vi "setUp.vi"(8 "error in (no error)":errorcluster, 11 "reference in":refnum<class "testcase-CSMNonCSMCallerSupportAPI.lvclass">) -> (0 "error out":errorcluster, 3 "reference out":refnum<class "testcase-CSMNonCSMCallerSupportAPI.lvclass">)   [LabVIEW 2017, in "testcase-CSMNonCSMCallerSupportAPI.lvclass"]
doc: "setUp runs prior to the test method during test execution. Use this method to initialize any object data required by your tests."
uses:
  testcase-CSMNonCSMCallerSupportAPI.lvclass
  C:/Program Files (x86)/National Instruments/LabVIEW 2017/vi.lib/addons/_JKI Toolkits/VI Tester/TestCase.llb/TestCase.lvclass
  testcase-CSMNonCSMCallerSupportAPI.lvclass/testcase-CSMNonCSMCallerSupportAPI.ctl
  <vilib>/addons/_JKI Toolkits/VI Tester/TestCase.llb/TestCase.lvclass
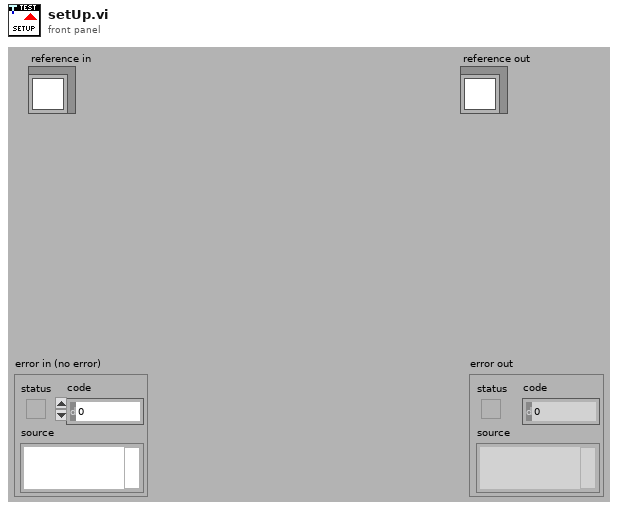
[diagram p1: front panel]
types:
  T1 = cluster{"name":string, "num":i32, "prototype":string[]}[]
  T2 = cluster{"prototype":string, "name":string, "num":i32, "index":i32}[]
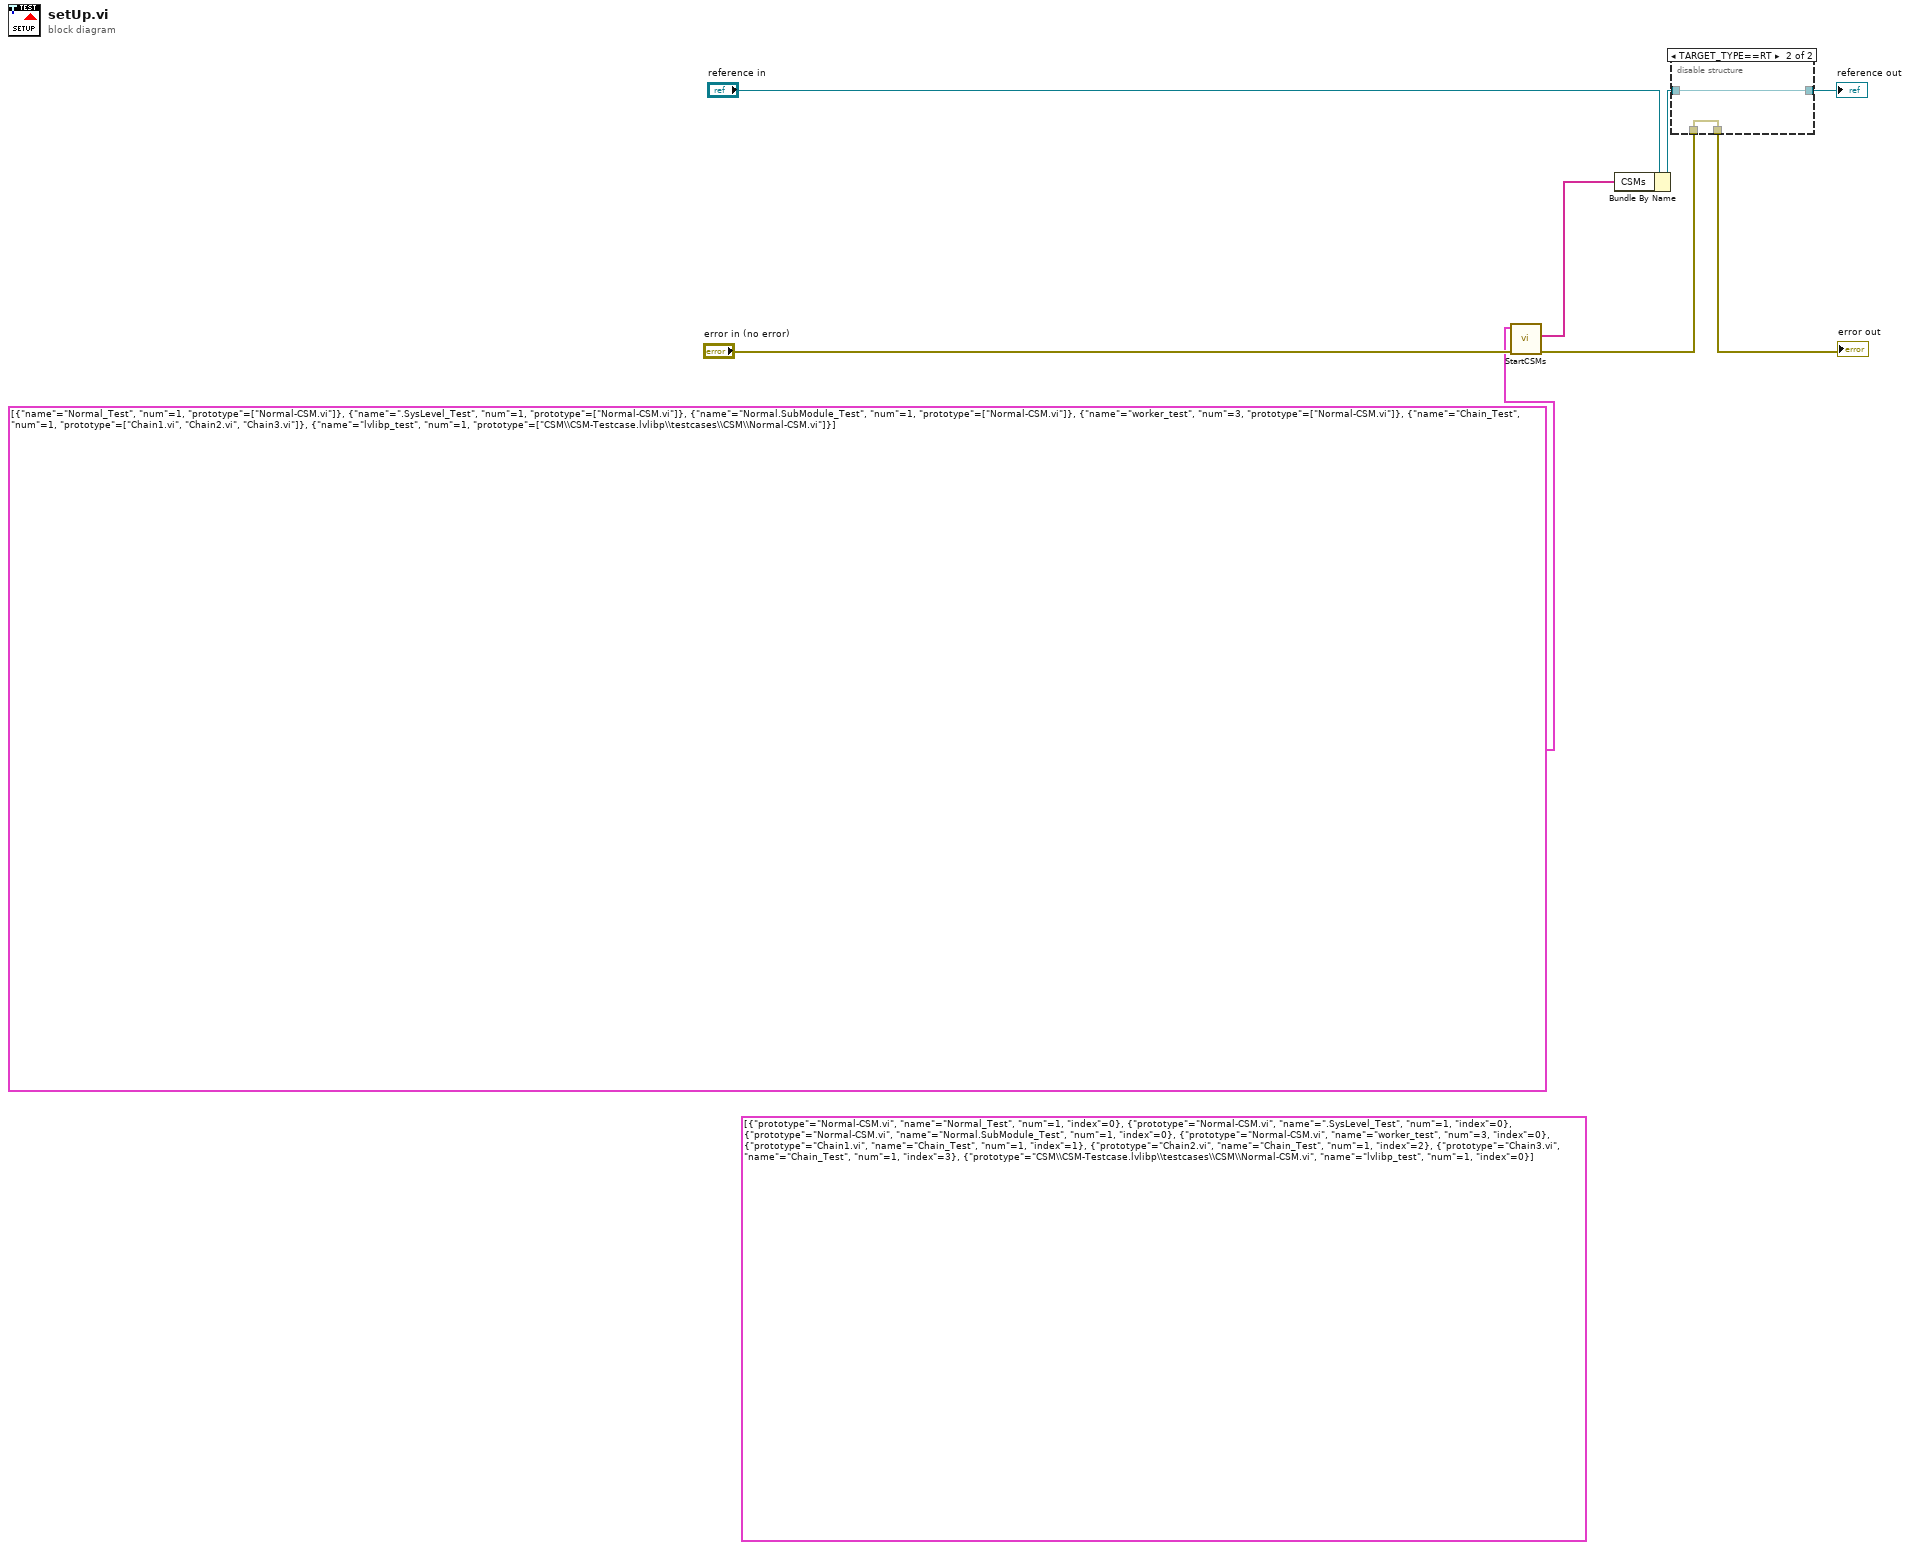
[diagram p0: block diagram]
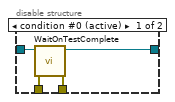
[diagram p2: hidden frame]
diagram:
  (unwired) T2 [{"prototype"="Normal-CSM.vi", "name"="Normal_Test", "num"=1, "index"=0}, {"prototype"="Normal-CSM.vi", "name"=".SysLevel_Test", "num"=1, "index"=0}, {"prototype"="Normal-CSM.vi", "name"="Normal.SubModule_Test", "num"=1, "index"=0}, {"prototype"="Normal-CSM.vi", "name"="worker_test", "num"=3, "index"=0}, {"prototype"="Chain1.vi", "name"="Chain_Test", "num"=1, "index"=1}, {"prototype"="Chain2.vi", "name"="Chain_Test", "num"=1, "index"=2}, {"prototype"="Chain3.vi", "name"="Chain_Test", "num"=1, "index"=3}, {"prototype"="CSM\\CSM-Testcase.lvlibp\\testcases\\CSM\\Normal-CSM.vi", "name"="lvlibp_test", "num"=1, "index"=0}]
  n1 = call "StartCSMs.vi"("error in"="error in (no error)", "Array"=T1 [{"name"="Normal_Test", "num"=1, "prototype"=["Normal-CSM.vi"]}, {"name"=".SysLevel_Test", "num"=1, "prototype"=["Normal-CSM.vi"]}, {"name"="Normal.SubModule_Test", "num"=1, "prototype"=["Normal-CSM.vi"]}, {"name"="worker_test", "num"=3, "prototype"=["Normal-CSM.vi"]}, {"name"="Chain_Test", "num"=1, "prototype"=["Chain1.vi", "Chain2.vi", "Chain3.vi"]}, {"name"="lvlibp_test", "num"=1, "prototype"=["CSM\\CSM-Testcase.lvlibp\\testcases\\CSM\\Normal-CSM.vi"]}]) -> ("error out"=w3:errorcluster, "CSMs"=w2:string[])  [unwired: 8 in]
  n2 = Bundle By Name(cluster="reference in", "CSMs"=w2) -> (w5:refnum<class "testcase-CSMNonCSMCallerSupportAPI.lvclass">)
  n3 = disable-structure shown="TARGET_TYPE==RT" {
    disable-tunnel: w3 -> [w12 w13]
    disable-tunnel: [w11 w13] -> w8
    disable-tunnel: [w10 w14] -> w6
    disable-tunnel: w5 -> [w9 w14]
    frame condition #0 (active) {
      n4 = call <vilib>:"WaitOnTestComplete.vi"("error in (no error)"=w12, "TestCase in"=w9) -> ("error out"=w11:errorcluster, "TestCase out"=w10:refnum<class "testcase-CSMNonCSMCallerSupportAPI.lvclass">)  [unwired: 8 in]
    }
    frame condition #1 {
    }
  }
  "error out" <- w8
  "reference out" <- w6
